vi "test_rm_depth_longthrow.vi"() -> ()   [LabVIEW 2023]
uses:
  <vilib>/picture/picture.llb/Draw True-Color Pixmap.vi
panel:
  out "Depth (modified)":picture
  out "AB (modified)":picture
  out "metadata":cluster{"sensor_ticks":u64}
  in  "host":string="192.168.1.7"
  in  "path in":path=path "C:/Users/jcds/Documents/GitHub/hl2ss/extensions/client_labview/hl2ss_labview/hl2ss_ulm.dll"
  in  "stop":bool
  out "pose":sgl[][](array[numeric])
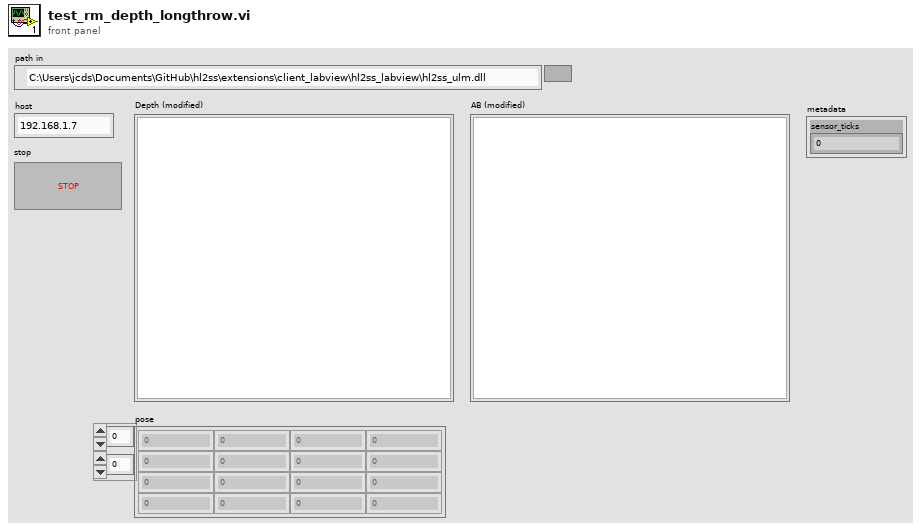
[diagram p1: front panel]
types:
  T1 = cluster{"chunk":u64, "mode":u8, "divisor":u8, "png_filter":u8, "_reserved_0":u8, "_reserved_1":u8, "_reserved_2":u8, "_reserved_3":u8, "_reserved_4":u8}
  T2 = cluster{"frame_stamp":i64, "timestamp":u64, "payload_size":u32, "status":i32, "payload":u64, "pose":u64}
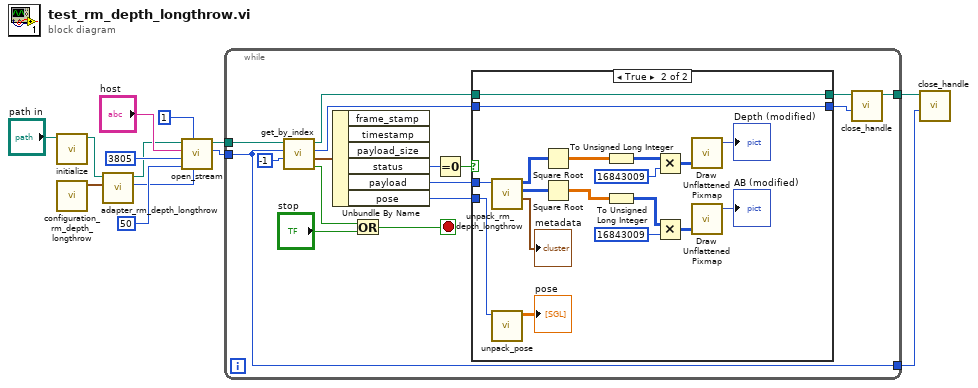
[diagram p0: block diagram]
diagram:
  n1 = call "initialize.vi"("path in"="path in") -> ("path out"=w4:path)  [unwired: 9 in, 1 out]
  n2 = call "configuration_rm_depth_longthrow.vi"() -> ("configuration_rm_depth_longthrow"=w5:T1)  [unwired: 11 in]
  n3 = call "adapter_rm_depth_longthrow.vi"("configuration_rm_depth_longthrow"=w5, "path in"=w4) -> ("configuration"=w2:u64, "path out"=w3:path)  [unwired: 8 in]
  n4 = call "open_stream.vi"("configuration"=w2, "decoded"=u8 1, "buffer_size"=u64 50, "port"=u16 3805, "host"="host", "path in"=w3) -> ("handle"=w13:u64, "path out"=w12:path)  [unwired: 3 in, 1 out]
  n5 = while {
    tunnel: [w20] -> w7
    tunnel: w13 -> [w14]
    tunnel: w12 -> [w15]
    tunnel: [w14] -> w6
    stop <- w19 stop-if-true
    n6 = call "get_by_index.vi"("frame_stamp"=i64 -1, "stream_handle"=w14, "path in"=w15) -> ("error"=w18:bool, "packet"=w29:T2, "packet_handle"=w23:u64, "path out"=w22:path)  [unwired: 5 in]
    n7 = Unbundle By Name(w29) -> ("status"=w28:i32, "payload"=w26:u64, "pose"=w25:u64)  [unwired: 3 out]
    n8 = Or(x=w18, y="stop") -> (x .or. y?=w19:bool)
    n9 = Equal To 0?(x=w28) -> (x = 0?=w27:bool)
    n10 = case shown="True" w27 {
      tunnel: w26 -> [_ w35]
      tunnel: w25 -> [_ w47]
      tunnel: [w30 w49] -> w24
      tunnel: w23 -> [w30 w49]
      tunnel: w22 -> [w31 w48]
      tunnel: [w31 w48] -> w21
      frame False {
      }
      frame True {
        n11 = call "unpack_rm_depth_longthrow.vi"("payload"=w35) -> ("metadata"=→"metadata":cluster{"sensor_ticks":u64}, "ab"=w33:u16[][], "depth"=w34:u16[][])  [unwired: 7 in, 1 out]
        n12 = call "unpack_pose.vi"("pose"=w47) -> ("pose"=→"pose":sgl[][])  [unwired: 9 in, 1 out]
        n13 = Square Root(x=w34) -> (sqrt(x)=w40:dbl[][])
        n14 = Square Root(x=w33) -> (sqrt(x)=w45:dbl[][])
        n15 = To Unsigned Long Integer(number=w40) -> (unsigned 32bit integer=w39:u32[][])
        n16 = To Unsigned Long Integer(number=w45) -> (unsigned 32bit integer=w44:u32[][])
        n17 = Multiply(x=w39, y=u32 16843009 ("frame_stamp")) -> (x*y=w37:u32[][])
        n18 = Multiply(x=w44, y=u32 16843009 ("frame_stamp")) -> (x*y=w42:u32[][])
        n19 = call-poly <vilib>:"Draw Unflattened Pixmap.vi"("data (RGB format)"=w37) -> ("new picture"=→"Depth (modified)":picture)  [unwired: 8 in]
        n20 = call-poly <vilib>:"Draw Unflattened Pixmap.vi"("data (RGB format)"=w42) -> ("new picture"=→"AB (modified)":picture)  [unwired: 8 in]
      }
    }
    n21 = call "close_handle.vi"("handle"=w24, "path in"=w21) -> ("path out"=w20:path)  [unwired: 9 in]
  }
  n22 = call "close_handle.vi"("handle"=w6, "path in"=w7) -> ()  [unwired: 9 in, 1 out]
